vi "写入天内各小时剂量数据.vi"(11 "设备终端.lvclass":refnum<class "设备终端.lvclass">) -> (3 "设备终端.o":refnum<class "设备终端.lvclass">)   [LabVIEW 2013, in "数据库操作.lvclass"]
uses:
  <vilib>/Utility/file.llb/Read From Spreadsheet File (string).vi
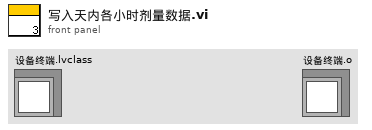
[diagram p1: front panel]
types:
  T1 = cluster{"用户名":string, "设备MAC":string, "设备状态":dbl, "密码":string, "职类":dbl, "姓名":string, "电话":string, "邮箱":string, "备注":string, "最后活动":string}
  T2 = typedef "NI_Database_API.lvlib/Conn ObjectReference.ctl" = refnum<k1>
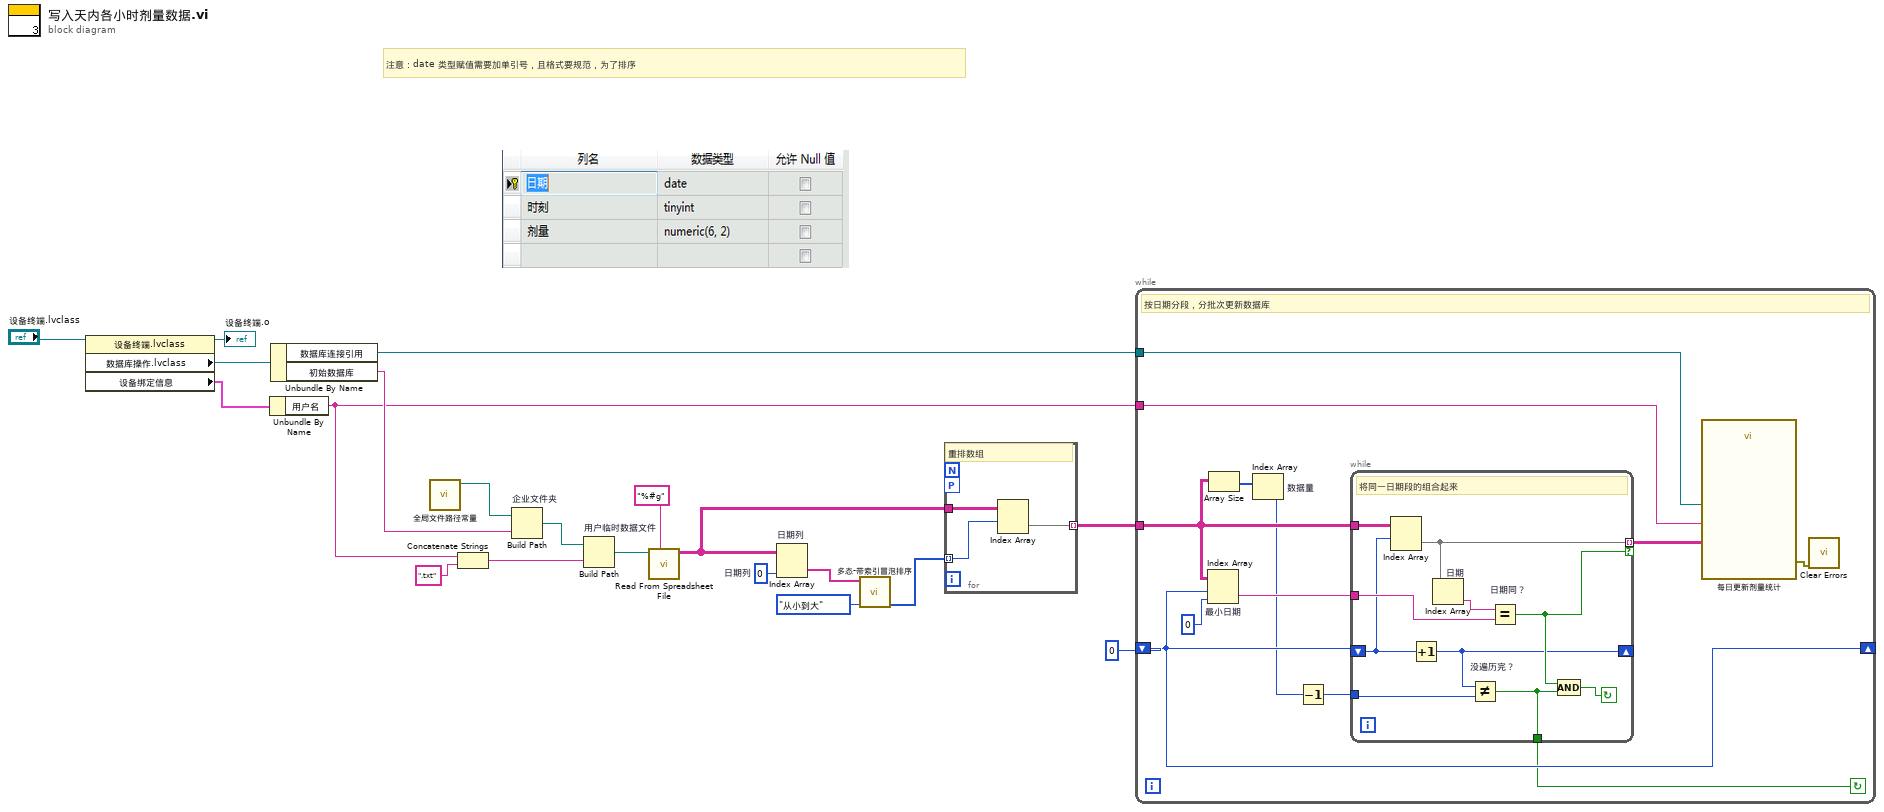
[diagram p0: block diagram]
diagram:
  w9 = 0  # 日期列
  # "注意：date 类型赋值需要加单引号，且格式要规范，为了排序"
  n1 = property class="设备终端.lvclass"(reference="设备终端.lvclass") -> (reference out=→"设备终端.o":refnum<class "设备终端.lvclass">, "数据库操作.lvclass"=w19:refnum<class "数据库操作.lvclass">, "设备绑定信息"=w18:T1)  [unwired: 1 in, 1 out]
  n2 = Unbundle By Name(w18) -> ("用户名"=w1:string)
  n3 = Unbundle By Name(w19) -> ("数据库连接引用"=w2:T2, "初始数据库"=w16:string)
  n4 = call "全局文件路径常量.vi"() -> ("用户数据库根目录"=w17:path)  [unwired: 9 in, 2 out]
  n5 = Concatenate Strings(w1, ".txt" ("字符串")) -> (w14:string)
  n6 = Build Path "企业文件夹"(base path=w17, name or relative path=w16) -> (appended path=w15:path)
  n7 = Build Path "用户临时数据文件"(base path=w15, name or relative path=w14) -> (appended path=w12:path)
  n8 = call-poly <vilib>:"Read From Spreadsheet File.vi"("format (%s)"="%#g", "file path (dialog if empty)"=w12) -> ("all rows"=w6:string[][])  [unwired: 5 in, 4 out]
  n9 = Index Array "日期列"(array=w6, index (col)=w9) -> (element=w8:string[])  [unwired: 1 in]
  n10 = call-poly "多态-带索引冒泡排序.vi"("排序模式"=enum16{"从小到大", "从大到小"}."从小到大", "数组"=w8) -> ("索引映射"=w5:i32[])  [unwired: 8 in, 1 out]
  n11 = for {
    tunnel: w5 -> [w23] mode=indexing
    tunnel: [w22] -> w4 mode=indexing
    workers-P: _ -> [_]
    tunnel: w6 -> [w21]
    # "重排数组"
    n12 = Index Array(array=w21, index (row)=w23) -> (element=w22:string[])  [unwired: 1 in]
  }
  n13 = while {
    tunnel: w4 -> [w33]
    shift-right: [w31] -> _
    shift-left: 0 -> [w31]
    tunnel: w2 -> [w29]
    tunnel: w1 -> [w28]
    stop <- w25 continue-if-true
    # "按日期分段，分批次更新数据库"
    n14 = Index Array "最小日期"(array=w33, index (row)=w31, index (col)=0 ("索引 (行)")) -> (element=w32:string)
    n15 = Array Size(array=w33) -> (size(s)=w34:i32[])
    n16 = Index Array "数据量"(array=w34) -> (element=w27:i32)  [unwired: 1 in]
    n17 = Decrement(x=w27) -> (x-1=w26:i32)
    n18 = while {
      tunnel: w33 -> [w45]
      shift-right: [w39] -> _
      shift-left: w31 -> [w40]
      tunnel: [w44] -> w30 mode=indexing if=w41
      tunnel: w32 -> [w42]
      tunnel: w26 -> [w38]
      tunnel: [w36] -> w25
      stop <- w37 continue-if-true
      # "将同一日期段的组合起来"
      n19 = Index Array(array=w45, index (row)=w40) -> (element=w44:string[])  [unwired: 1 in]
      n20 = Increment(x=w40) -> (x+1=w39:i32)
      n21 = Index Array "日期"(array=w44) -> (element=w43:string)  [unwired: 1 in]
      n22 = Not Equal? "没遍历完？"(x=w39, y=w38) -> (x != y?=w36:bool)
      n23 = Equal? "日期同？"(x=w43, y=w42) -> (x = y?=w41:bool)
      n24 = Compound Arithmetic op=AND(w41, w36) -> (w37:bool)
    }
    n25 = call "每日更新剂量统计.vi"("天内数据"=w30, "用户名"=w28, "数据库连接引用"=w29) -> ("error out"=w24:errorcluster)  [unwired: 8 in]
    n26 = call <vilib>:"Clear Errors.vi"("error in (no error)"=w24) -> ()  [unwired: 6 in, 1 out]
  }
